vi "Edit Config.vi"(8 "error in (no error)":errorcluster, 11 "NI DA in":refnum<class "NI Digital to Analog.lvclass">) -> (0 "error out":errorcluster, 3 "NI DA out":refnum<class "NI Digital to Analog.lvclass">)   [LabVIEW 2018, in "NI Digital to Analog.lvclass"]
doc: "NI Analog.lvclass:Edit Config.vi\n\nThis VI is used to edit the NI Analog configuration parameters.\n\nInstrument Communication Module Version 1.0\nJanuary, 2018 Original Code Consulting David Thomson\n www.originalcode.com"
uses:
  NI Digital to Analog.lvclass
  NI Analog Config.ctl
  NI Analog Channel Range.ctl
  ICM Class Editor State.ctl
  ICM Editor Command.ctl
  NI Digital to Analog.lvclass/NI Digital to Analog.ctl
panel:
  out "Device Table":string[][](table)
  in  "Flash Save":bool
  in  "Save":bool
  in  "Revert":bool
  in  "NI DA Config":T1
  # "This bus must use the\nNo-Op output"
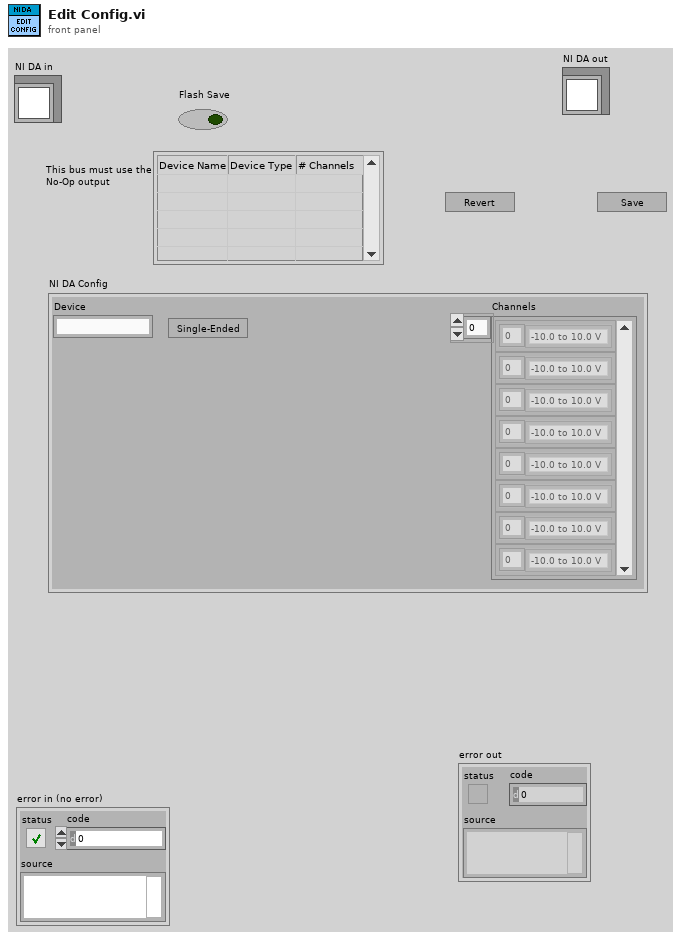
[diagram p1: front panel]
types:
  T1 = typedef "NI Analog Config.ctl" = cluster{"Device":string, "SE/Diff":bool, "Channels":cluster{"Channel":i32, "Range":T2}[]}
  T2 = typedef "NI Analog Channel Range.ctl" = enum16{"-10.0 to 10.0 V", "-5.0 to 5.0 V", "-2.0 to 2.0 V", "-1.0 to 1.0 V", "-0.5 to 0.5 V", "-0.2 to 0.2 V", "-0.1 to 0.1 V", "0 to 10 V", "0 to 5 V", "0 to 2 V", "0 to 1 V", "0 to 0.5 V", "0 to 0.2 V", "0 to 0.1 V"}
  T3 = typedef "ICM Editor Command.ctl" = enum16{"No-op", "Exit"}
  T4 = typedef "ICM Class Editor State.ctl" = enum16{"Init", "Wait", "Write", "Read", "Display", "Set Flashing", "Error", "Stop"}
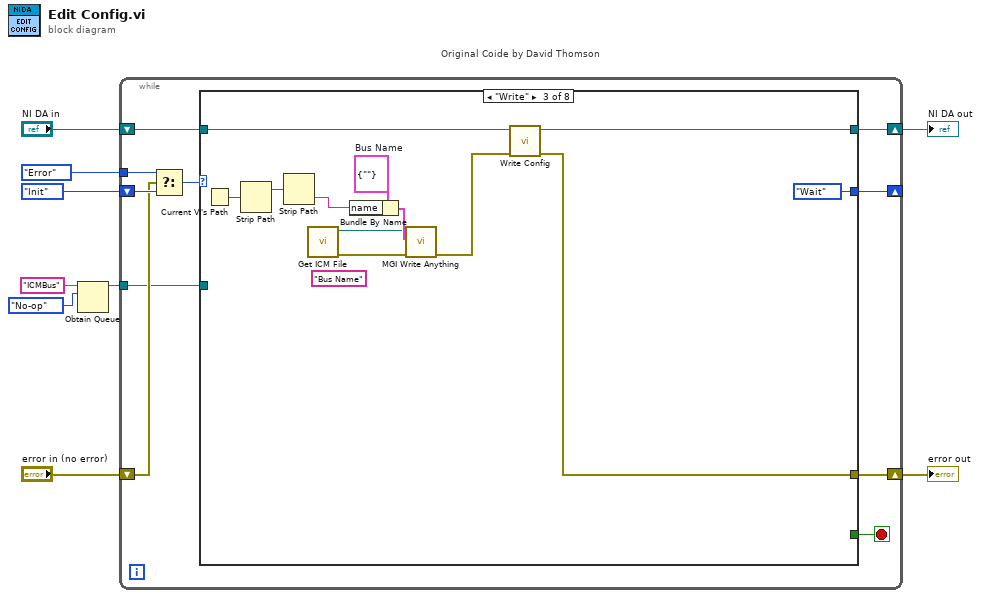
[diagram p0: block diagram]
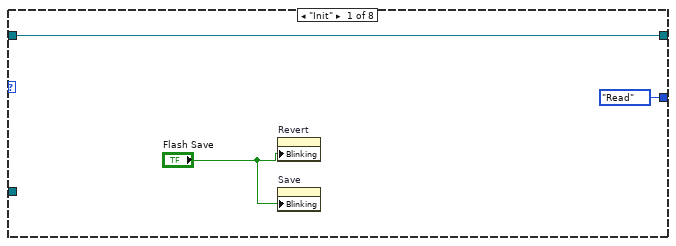
[diagram p2: hidden frame]
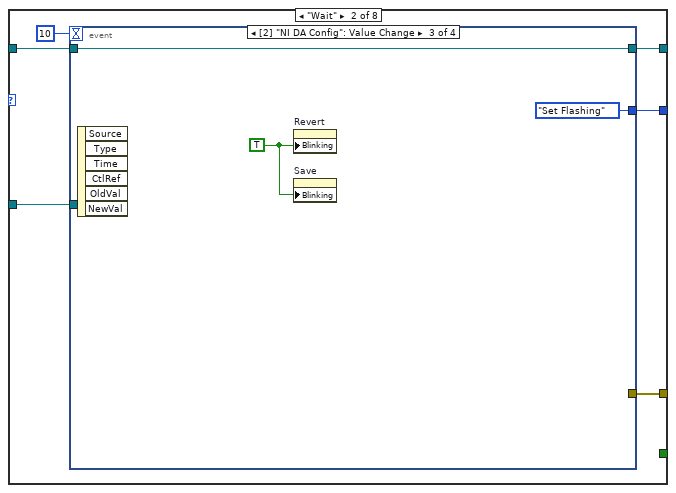
[diagram p3: hidden frame]
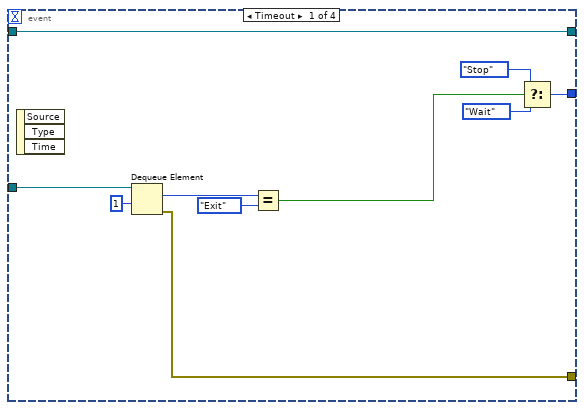
[diagram p4: hidden frame]
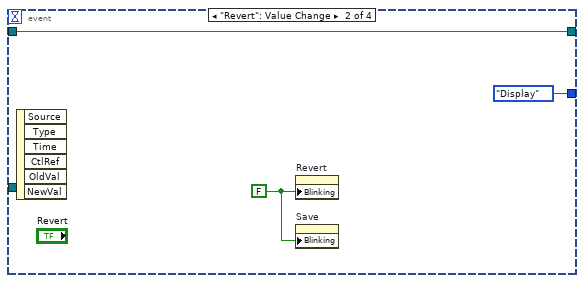
[diagram p5: hidden frame]
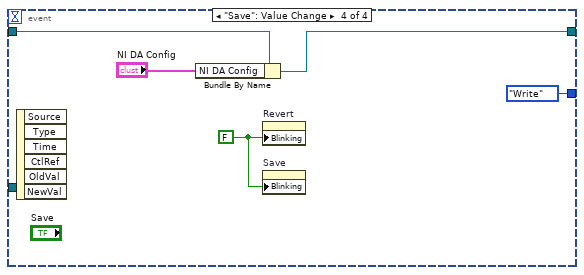
[diagram p6: hidden frame]
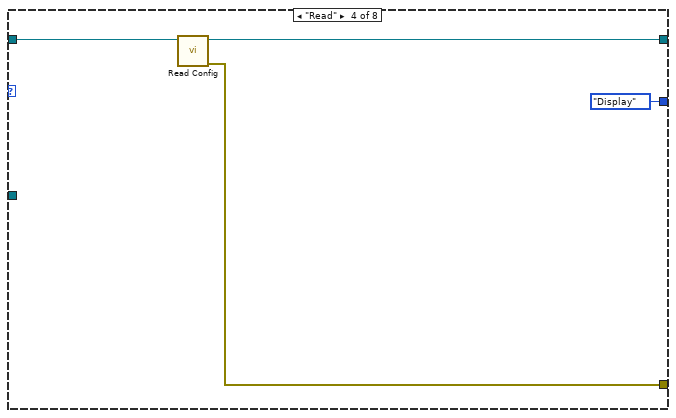
[diagram p7: hidden frame]
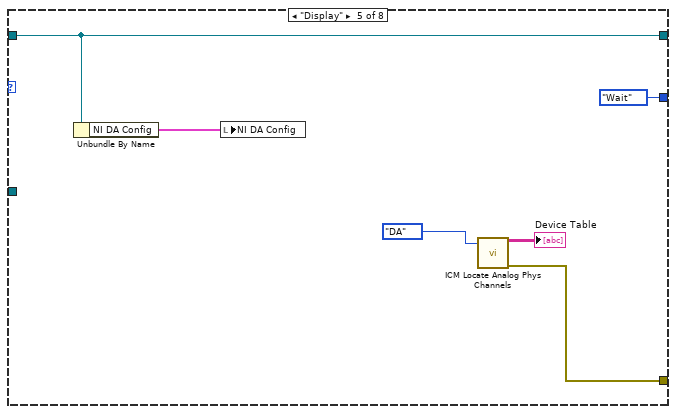
[diagram p8: hidden frame]
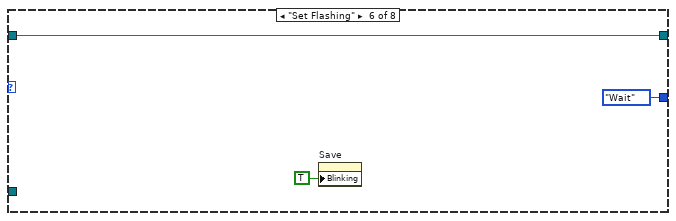
[diagram p9: hidden frame]
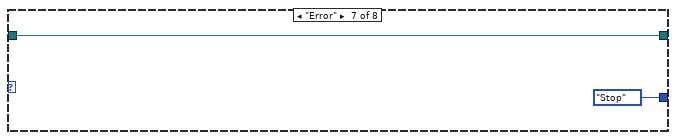
[diagram p10: hidden frame]
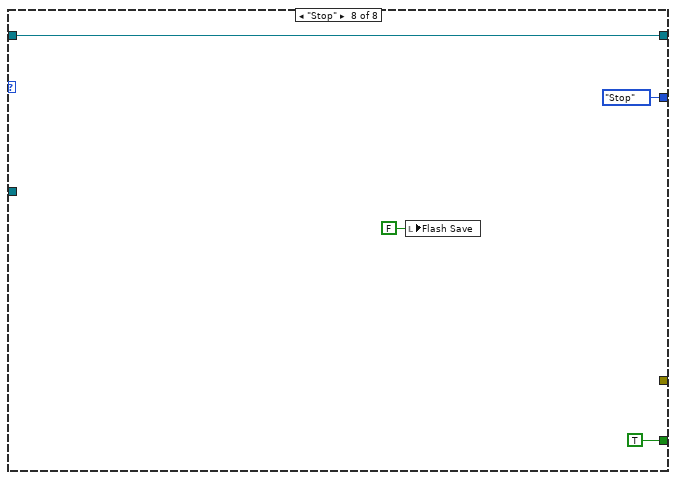
[diagram p11: hidden frame]
diagram:
  n1 = Obtain Queue(name (unnamed)="ICMBus", element data type=ICM_Editor_Command."No-op" ("Editor Command")) -> (queue out=w1:refnum<queue>)  [unwired: 3 in, 2 out]
  n2 = while "Original Coide by David Thomson" {
    shift-right: [w19] -> w8
    shift-left: "NI DA in" -> [w18]
    shift-right: [w12] -> _
    shift-left: ICM_Class_Editor_State."Init" ("Config State") -> [w16]
    shift-right: [w11] -> w6
    shift-left: "error in (no error)" -> [w14]
    tunnel: ICM_Class_Editor_State."Error" ("Config State") -> [w13]
    tunnel: w1 -> [w10]
    stop <- w17 stop-if-true
    n3 = Select(t=w13, s=w14, f=w16) -> (s? t:f=w15:T4)
    n4 = case shown="\"Write\"" w15 {
      tunnel: [w21 w26 w59 w63 w71 w74 w76 w80] -> w19
      tunnel: w18 -> [w21 w25 w60 w65 w71 w74 w76 w80]
      tunnel: [_ _ _ _ _ _ _ TRUE] -> w17
      tunnel: [ICM_Class_Editor_State."Read" ("Config State") w27 ICM_Class_Editor_State."Wait" ("Config State") ICM_Class_Editor_State."Display" ("Config State") ICM_Class_Editor_State."Wait" ("Config State") ICM_Class_Editor_State."Wait" ("Config State") ICM_Class_Editor_State."Stop" ("Config State") ICM_Class_Editor_State."Stop" ("Config State")] -> w12
      tunnel: [_ w23 w58 w64 w67 _ _ _] -> w11
      tunnel: w10 -> [_ w24 _ _ _ _ _ _]
      frame "Init" {
        n5 = property on="Revert" class="Bool"("Blinking"="Flash Save") -> ()  [unwired: 2 in, 2 out]
        n6 = property on="Save" class="Bool"("Blinking"="Flash Save") -> ()  [unwired: 2 in, 2 out]
      }
      frame "Wait" {
        n7 = event shown="[2] \"NI DA Config\": Value Change" {
          selector: _ -> [_ _ _ _]
          dyn-events: _ -> [_ _ _ _]
          timeout: 10 -> [_ _ _ _]
          tunnel: [w35 ICM_Class_Editor_State."Display" ("Config State") ICM_Class_Editor_State."Set Flashing" ("Config State") ICM_Class_Editor_State."Write" ("Config State")] -> w27
          tunnel: [w38 w40 w44 w46] -> w26
          tunnel: w25 -> [w38 w40 w44 w47]
          tunnel: w24 -> [w37 _ _ _]
          tunnel: [w29 _ _ _] -> w23
          event Timeout {
            n8 = event-data() -> ()  [unwired: 1 in, 3 out]
            n9 = Dequeue Element(queue=w37, timeout in ms (-1)=1) -> (element=w34:T3, error out=w29:errorcluster)  [unwired: 1 in, 2 out]
            n10 = Equal?(x=w34, y=ICM_Editor_Command."Exit") -> (x = y?=w32:bool)
            n11 = Select(t=ICM_Class_Editor_State."Stop" ("Config State"), s=w32, f=ICM_Class_Editor_State."Wait" ("Config State")) -> (s? t:f=w35:T4)
          }
          event "Revert": Value Change {
            w39 = FALSE ("Blinking")
            n12 = event-data() -> ()  [unwired: 1 in, 6 out]
            n13 = property on="Revert" class="Bool"("Blinking"=w39) -> ()  [unwired: 2 in, 2 out]
            n14 = property on="Save" class="Bool"("Blinking"=w39) -> ()  [unwired: 2 in, 2 out]
          }
          event Value Change {
            w42 = TRUE ("Blinking")
            n15 = event-data() -> ()  [unwired: 1 in, 6 out]
            n16 = property on="Revert" class="Bool"("Blinking"=w42) -> ()  [unwired: 2 in, 2 out]
            n17 = property on="Save" class="Bool"("Blinking"=w42) -> ()  [unwired: 2 in, 2 out]
          }
          event "Save": Value Change {
            w45 = FALSE ("Blinking")
            n18 = event-data() -> ()  [unwired: 1 in, 6 out]
            n19 = Bundle By Name(cluster=w47, "NI DA Config"="NI DA Config") -> (w46:refnum<class "NI Digital to Analog.lvclass">)
            n20 = property on="Revert" class="Bool"("Blinking"=w45) -> ()  [unwired: 2 in, 2 out]
            n21 = property on="Save" class="Bool"("Blinking"=w45) -> ()  [unwired: 2 in, 2 out]
          }
        }
      }
      frame "Write" {
        w54 = cluster{"name":string} {"name"=""}  # Bus Name
        (unwired) "Bus Name" ("Section Name (Name of \"Anything\")")
        n22 = Current VI's Path() -> (path=w57:path)
        n23 = Strip Path(path=w57) -> (stripped path=w56:path)  [unwired: 1 out]
        n24 = Strip Path(path=w56) -> (name=w53:string)  [unwired: 1 out]
        n25 = call "Get ICM File.vi"() -> ("error out"=w55:errorcluster, "ICM File"=w50:path)  [unwired: 10 in]
        n26 = Bundle By Name(cluster=w54, "name"=w53) -> (w52:cluster{"name":string})
        n27 = call "MGI Write Anything.vi"("Error In"=w55, "Anything"=w52, "Path (dialog)"=w50) -> ("Error Out"=w51:errorcluster)  [unwired: 6 in, 2 out]
        n28 = call-dynamic "Write Config.vi"("error in (no error)"=w51, "NI DA in"=w60) -> ("error out"=w58:errorcluster, "NI DA out"=w59:refnum<class "NI Digital to Analog.lvclass">)  [unwired: 8 in]
      }
      frame "Read" {
        n29 = call-dynamic "Read Config.vi"("NI DA in"=w65) -> ("error out"=w64:errorcluster, "NI DA out"=w63:refnum<class "NI Digital to Analog.lvclass">)  [unwired: 9 in]
      }
      frame "Display" {
        n30 = Unbundle By Name(w71) -> ("NI DA Config"=w70:T1)
        n31 = local write "NI DA Config"(w70) -> ()
        n32 = call "ICM Locate Analog Phys Channels.vi"("Channel Type"=enum16{"AD SE", "AD Diff", "DA"}."DA") -> ("Table"=→"Device Table":string[][], "error out"=w67:errorcluster)  [unwired: 13 in]
      }
      frame "Set Flashing" {
        n33 = property on="Save" class="Bool"("Blinking"=TRUE) -> ()  [unwired: 2 in, 2 out]
      }
      frame "Error" {
      }
      frame "Stop" {
        n34 = local write "Flash Save"(FALSE ("Flash Save")) -> ()
      }
    }
  }
  "error out" <- w6
  "NI DA out" <- w8
